vi "Fy_Gravity_compensation.vi"(10 "AbsolutePositionRotation in":dbl, 11 "Fy_to_filter":dbl) -> (2 "Gravity compensation":dbl(graph), 3 "F_y[N] Gravity compensated 2":dbl(graph))   [LabVIEW 2019]
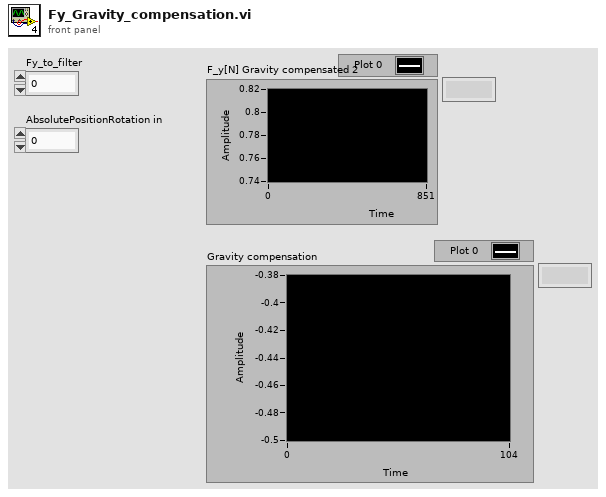
[diagram p1: front panel]
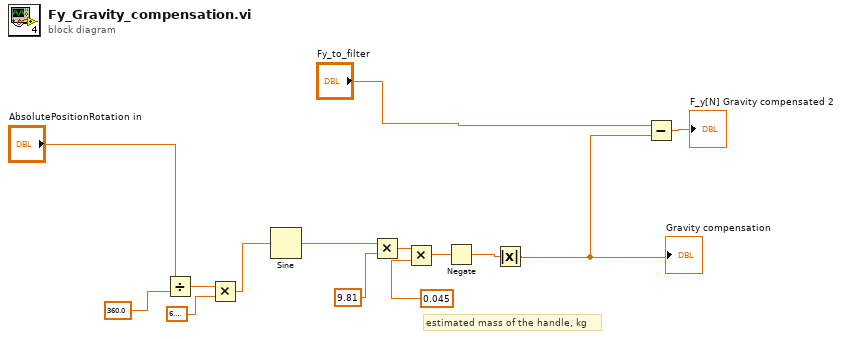
[diagram p0: block diagram]
diagram:
  # "estimated mass of the handle, kg"
  n1 = Divide(x="AbsolutePositionRotation in", y=360.0) -> (x/y=w7:dbl)
  n2 = Multiply(x=w7, y=6.283185307179586) -> (x*y=w9:dbl)
  n3 = Sine(x=w9) -> (sin(x)=w10:dbl)
  n4 = Multiply(x=w10, y=9.81) -> (x*y=w11:dbl)
  n5 = Multiply(x=w11, y=0.045 ("mass")) -> (x*y=w14:dbl)
  n6 = Negate(x=w14) -> (-x=w2:dbl)
  n7 = Absolute Value(x=w2) -> (abs(x)=w1:dbl)
  "Gravity compensation" <- w1
  n8 = Subtract(x="Fy_to_filter", y=w1) -> (x-y=→"F_y[N] Gravity compensated 2":dbl)
